vi "TIO SLIP Decode.vi"(2 "error in (no error)":errorcluster, 3 "SLIP Input":string="\u00124VxÛ\u0000") -> (0 "error out":errorcluster, 1 "String Output":string)   [LabVIEW 2020]
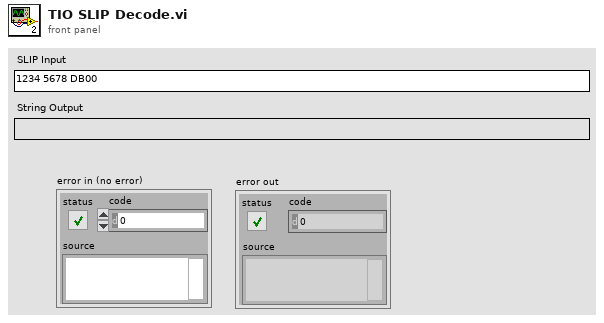
[diagram p1: front panel]
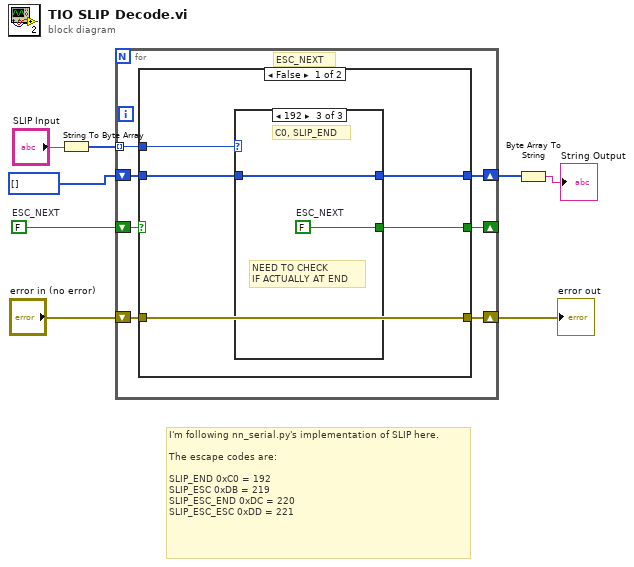
[diagram p0: block diagram]
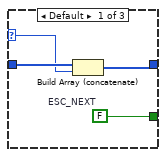
[diagram p2: hidden frame]
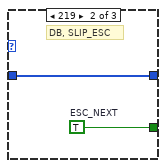
[diagram p3: hidden frame]
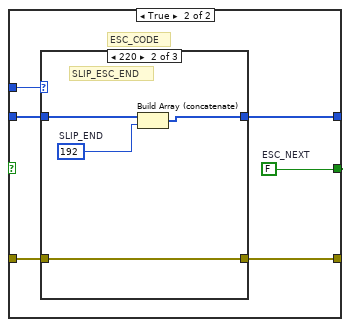
[diagram p4: hidden frame]
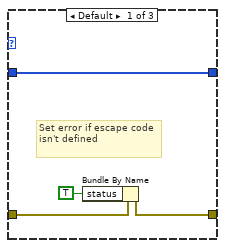
[diagram p5: hidden frame]
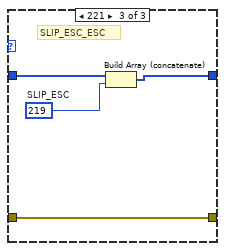
[diagram p6: hidden frame]
diagram:
  w4 = FALSE  # ESC_NEXT
  # "I'm following nn_serial.py's implementation of SLIP here. \n\nThe escape codes are:\n\nSLIP_END\t0xC0 = 192\nSLIP_ESC\t0xDB = 219\nSLIP_ESC_END\t0xDC = 220\nSLIP_ESC_ESC\t0xDD = 221"
  n1 = String To Byte Array(string="SLIP Input") -> (unsigned byte array=w7:u8[])
  n2 = for {
    tunnel: w7 -> [w13] mode=indexing
    shift-right: [w14] -> w1
    shift-left: u8[] [] ("unsigned byte array") -> [w15]
    shift-right: [w12] -> _
    shift-left: w4 -> [w11]
    shift-right: [w9] -> w2
    shift-left: "error in (no error)" -> [w10]
    # "ESC_NEXT"
    n3 = case shown="False" w11 {
      tunnel: w15 -> [w20 w34]
      tunnel: [w19 w33] -> w14
      tunnel: w13 -> [w17 w32]
      tunnel: [w18 w31] -> w12
      tunnel: w10 -> [w16 w30]
      tunnel: [w16 w29] -> w9
      frame False {
        n4 = case shown="192" w17 {
          selector: w17 -> [w23 _ _]
          tunnel: w20 -> [w24 w26 w28]
          tunnel: [w22 w26 w28] -> w19
          tunnel: [w21 w25 w27] -> w18
          frame Default {
            w21 = FALSE  # ESC_NEXT
            n5 = Build Array (concatenate)(w24, w23) -> (w22:u8[])
          }
          frame 219 {
            w25 = TRUE  # ESC_NEXT
            # "DB, SLIP_ESC"
          }
          frame 192 {
            w27 = FALSE  # ESC_NEXT
            # "NEED TO CHECK\nIF ACTUALLY AT END"
            # "C0, SLIP_END"
          }
        }
      }
      frame True {
        w31 = FALSE  # ESC_NEXT
        # "ESC_CODE"
        n6 = case shown="220" w32 {
          tunnel: w34 -> [w35 w41 w45]
          tunnel: [w35 w40 w44] -> w33
          tunnel: w30 -> [w38 w39 w43]
          tunnel: [w37 w39 w43] -> w29
          frame Default {
            # "Set error if escape code isn't defined"
            n7 = Bundle By Name(cluster=w38, "status"=TRUE) -> (w37:errorcluster)
          }
          frame 220 {
            w42 = u8 192  # SLIP_END
            # "SLIP_ESC_END"
            n8 = Build Array (concatenate)(w41, w42) -> (w40:u8[])
          }
          frame 221 {
            w46 = u8 219  # SLIP_ESC
            # "SLIP_ESC_ESC"
            n9 = Build Array (concatenate)(w45, w46) -> (w44:u8[])
          }
        }
      }
    }
  }
  "error out" <- w2
  n10 = Byte Array To String(unsigned byte array=w1) -> (string=→"String Output":string)
